vi "FRC-Traj-Lib-SlewRateLimiter-Sample.vi"() -> ()   [LabVIEW 2019]
uses:
  <vilib>/Rock Robotics/WPI/ThirdParty/JAS_Junk/TrajLib/Trajectory_Library.lvlib
panel:
  in  "Tab Control":enum32{"Control Panel", "Logic"}(tab)
  out "Output 1":dbl
  in  "Rate Limit":dbl=10.0
  in  "Input":dbl(slide)=10.0 scale=-100.0..100.0
  out "Output 2":dbl
  in  "Enable":bool
  out "Trend":cluster{dbl, dbl, "Value_Output":dbl}(graph)
  out "Enabled":bool
  # "SlewRateLimiter Sample"
  # "Rate Limited"
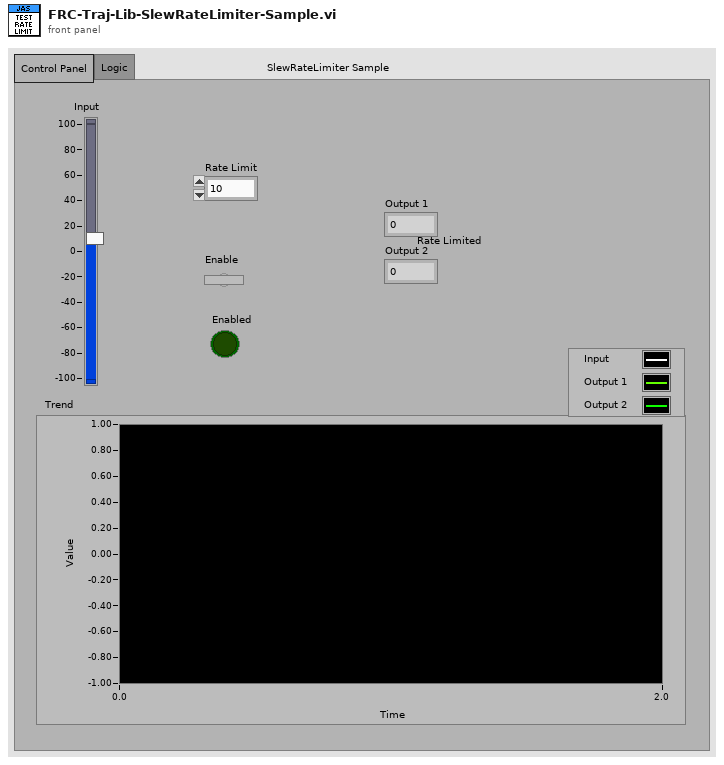
[diagram p1: front panel]
types:
  T1 = typedef "Trajectory_Library.lvlib/SLEW_RATE_LIMITER.ctl" = cluster{"RateLimit":dbl, "PrevValue":dbl, "PrevTime":dbl}
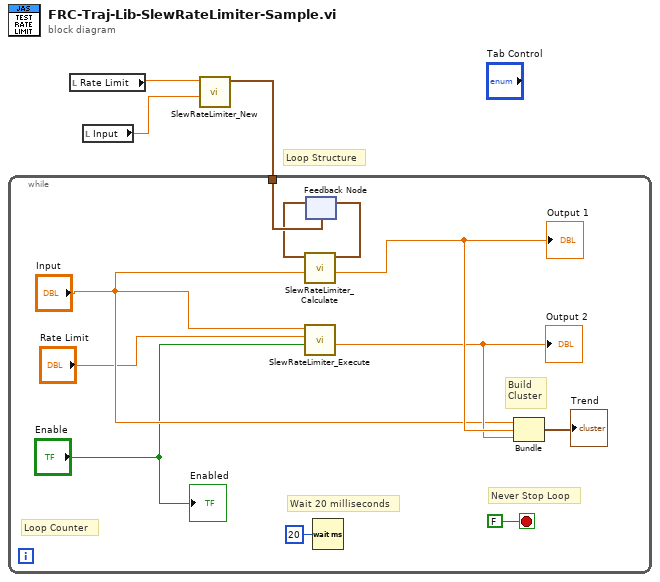
[diagram p0: block diagram]
diagram:
  # "Loop Structure"
  n1 = local read "Rate Limit"() -> (w1:dbl)
  n2 = local read "Input"() -> (w2:dbl)
  n3 = call <vilib>:"SlewRateLimiter_New.vi"("InitialValue"=w2, "RateLimit"=w1) -> ("out SLEW_RATE_LIMITER"=w3:T1)  [unwired: 9 in]
  n4 = while {
    tunnel: w3 -> [w11]
    stop <- FALSE stop-if-true
    # "Build\nCluster"
    # "Loop Counter"
    # "Never Stop Loop"
    # "Wait 20 milliseconds"
    n5 = call <vilib>:"SlewRateLimiter_Execute.vi"("Enable"="Enable", "Rate"="Rate Limit", "Input"="Input") -> ("Output"=w7:dbl)  [unwired: 7 in, 1 out]
    "Output 2" <- w7
    n6 = feedback #1(w11) -> (w10:T1)
    n7 = call <vilib>:"SlewRateLimiter_Calculate.vi"("Input"="Input", "in SLEW_RATE_LIMITER"=w10) -> ("Output"=w8:dbl, "out SLEW_RATE_LIMITER"=w9:T1)  [unwired: 8 in]
    "Output 1" <- w8
    n8 = feedback-in #1(w9) -> ()
    n9 = Wait (ms)(milliseconds to wait=u32 20) -> ()  [unwired: 1 out]
    n10 = Bundle("Input"="Input", "Output"=w8, "Output"=w7) -> (→"Trend":cluster{"Input":dbl, "Output":dbl, "Output":dbl})  [unwired: 1 in]
    "Enabled" <- "Enable"
  }
